vi "Display Configuration.vi"() -> ()   [LabVIEW 2014]
uses:
  Typedef/State_PCMonitors_Configuration.ctl
  <vilib>/Utility/config.llb/NI_LVConfig.lvlib
  <vilib>/Utility/config.llb/Read Key (String).vi
  <vilib>/Utility/config.llb/Write Key (String).vi
panel:
  out "PC name":string
  in  "Path":path
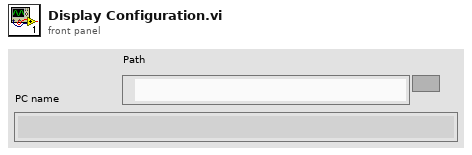
[diagram p1: front panel]
types:
  T1 = typedef "State_PCMonitors_Configuration.ctl" = enum16{"File exist", "Check PC ", "Create config file"}
  T2 = typedef "NI_LVConfig.lvlib/Config Data RefNum.ctl" = refnum<k1>
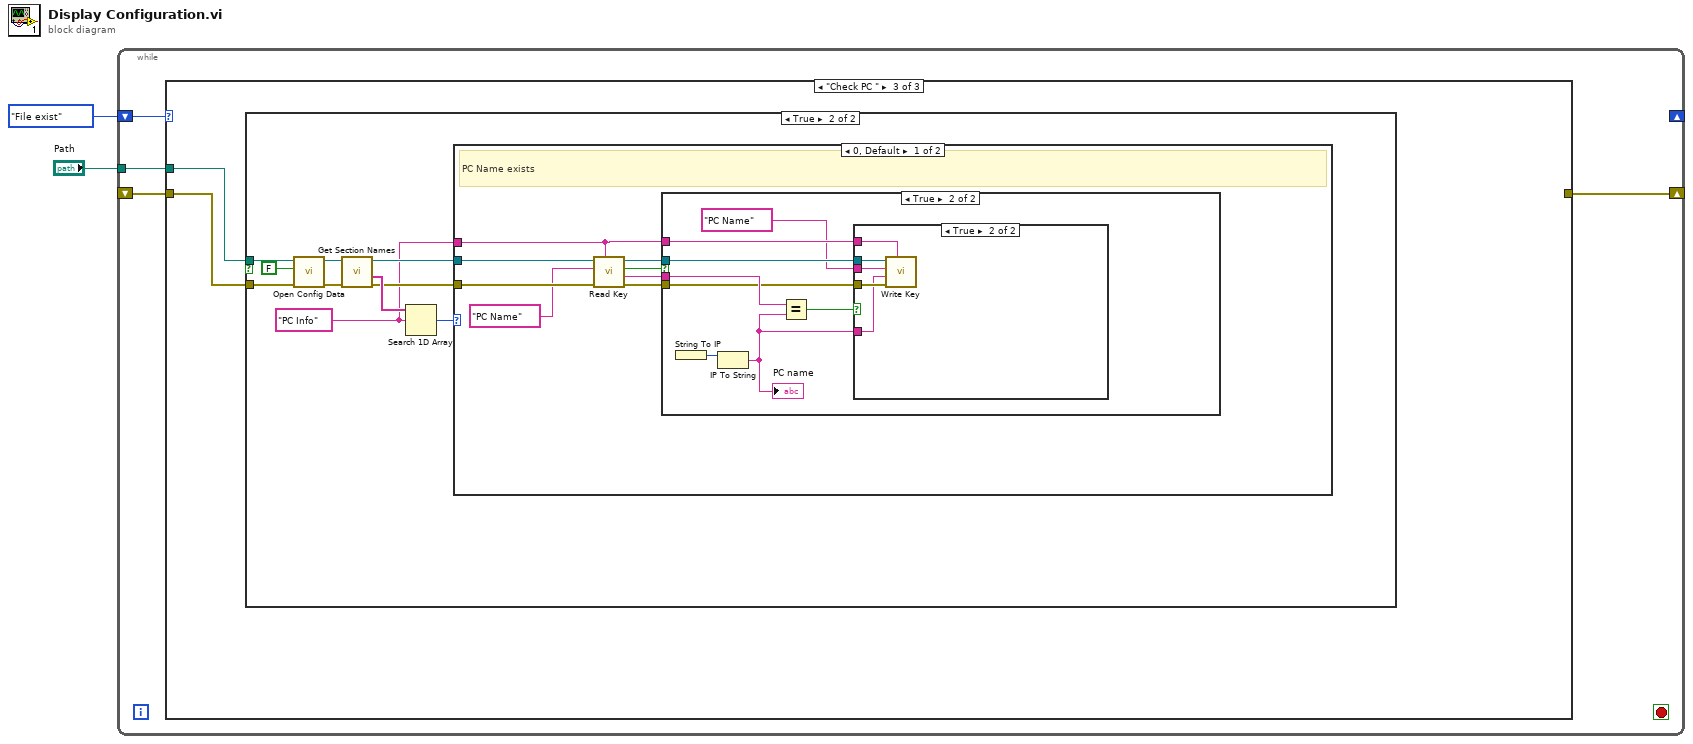
[diagram p0: block diagram]
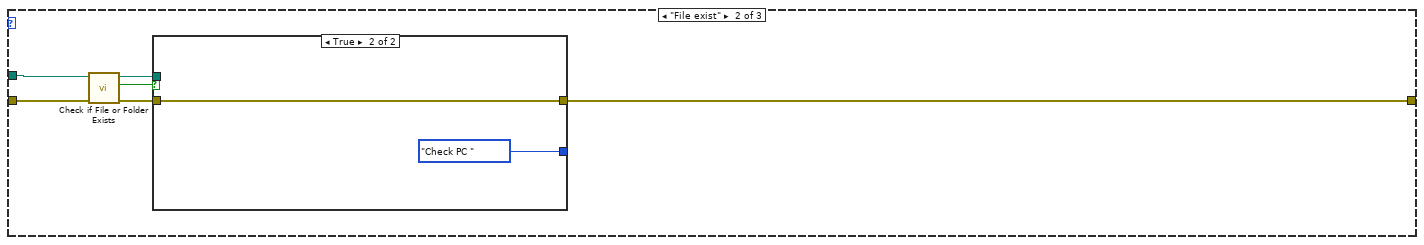
[diagram p3: hidden frame]
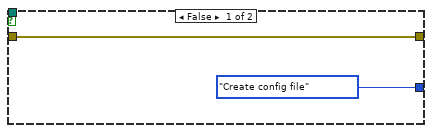
[diagram p4: hidden frame]
diagram:
  n1 = while {
    shift-right: _ -> [_]
    shift-left: State_PCMonitors_Configuration."File exist" -> [w6]
    tunnel: "Path" -> [w5]
    shift-right: [w3] -> _
    shift-left: _ -> [w4]
    stop <- _ stop-if-true
    n2 = case shown="\"Check PC \"" w6 {
      tunnel: w5 -> [_ w12 w18]
      tunnel: w4 -> [_ w11 w17]
      tunnel: [_ w7 _] -> w3
      frame "File exist" {
      }
      frame "File exist" {
        n3 = call <vilib>:"Check if File or Folder Exists.vi"("error in (no error)"=w11, "path"=w12) -> ("error out"=w9:errorcluster, "file or folder exists?"=w10:bool, "dup path"=w8:path)  [unwired: 7 in]
        n4 = case shown="True" w10 {
          tunnel: w9 -> [w14 w15]
          tunnel: w8 -> [_ _]
          tunnel: [State_PCMonitors_Configuration."Create config file" State_PCMonitors_Configuration."Check PC "] -> _
          tunnel: [w14 w15] -> w7
          frame False {
          }
          frame True {
          }
        }
      }
      frame "Check PC " {
        n5 = case shown="True" {
          selector: _ -> [_ _]
          tunnel: w17 -> [_ w27]
          tunnel: w18 -> [_ w28]
          frame False {
          }
          frame True {
            w19 = "PC Info" ("element")
            n6 = call <vilib>:"Open Config Data.vi"("error in (no error)"=w27, "create file if necessary (T)"=FALSE, "configuration file path"=w28) -> ("error out"=w25:errorcluster, "refnum"=w24:T2)  [unwired: 6 in, 1 out]
            n7 = call <vilib>:"Get Section Names.vi"("error in (no error)"=w25, "refnum"=w24) -> ("error out"=w20:errorcluster, "section names"=w23:string[], "refnum out"=w21:T2)  [unwired: 7 in]
            n8 = Search 1D Array(1D array=w23, element=w19) -> (index of element=w22:i32)  [unwired: 1 in]
            n9 = case shown="0, Default" w22 {
              tunnel: w21 -> [w36 _]
              tunnel: w20 -> [w35 _]
              tunnel: w19 -> [w29 _]
              frame 0, Default {
                # "PC Name exists"
                n10 = call-poly <vilib>:"Read Key.vi"("section"=w29, "error in (no error)"=w35, "key"="PC Name" ("element"), "refnum"=w36) -> ("error out"=w31:errorcluster, "value"=w34:string, "found?"=w32:bool, "refnum out"=w30:T2)  [unwired: 4 in]
                n11 = case shown="True" w32 {
                  tunnel: w34 -> [_ w43]
                  tunnel: w31 -> [_ w40]
                  tunnel: w30 -> [_ w41]
                  tunnel: w29 -> [_ w39]
                  frame False {
                  }
                  frame True {
                    n12 = String To IP() -> (0:w44:u32)  [unwired: 1 in]
                    n13 = IP To String(2:w44) -> (0:w37:string)  [unwired: 1 in]
                    "PC name" <- w37
                    n14 = Equal?(x=w43, y=w37) -> (x = y?=w42:bool)
                    n15 = case shown="True" w42 {
                      tunnel: w41 -> [_ w49]
                      tunnel: w40 -> [_ w48]
                      tunnel: w39 -> [_ w47]
                      tunnel: "PC Name" ("element") -> [_ w46]
                      tunnel: w37 -> [_ w45]
                      frame False {
                      }
                      frame True {
                        n16 = call-poly <vilib>:"Write Key.vi"("section"=w47, "error in (no error)"=w48, "value"=w45, "key"=w46, "refnum"=w49) -> ()  [unwired: 4 in, 3 out]
                      }
                    }
                  }
                }
              }
              frame -1 {
                # "PC Name does not exist"
              }
            }
          }
        }
      }
    }
  }
